vi "Information.vi"(8 "error in (no error)":errorcluster, 9 "Context":T1, 10 "Information":refnum<class "Information.lvclass">, 11 "Process Controller in":refnum<class "Process Controller.lvclass">) -> (0 "error out":errorcluster, 3 "Process Controller out":refnum<class "Process Controller.lvclass">)   [LabVIEW 2021, in "Process Controller.lvclass"]
uses:
  Process Controller.lvclass
  Publish-Subscribe/Interfaces/Information/Information.lvclass
  Publish-Subscribe/Context.ctl
  NHMFL_Core/Libraries/Instruments/Results/Acquired Result/Acquired Result.lvclass
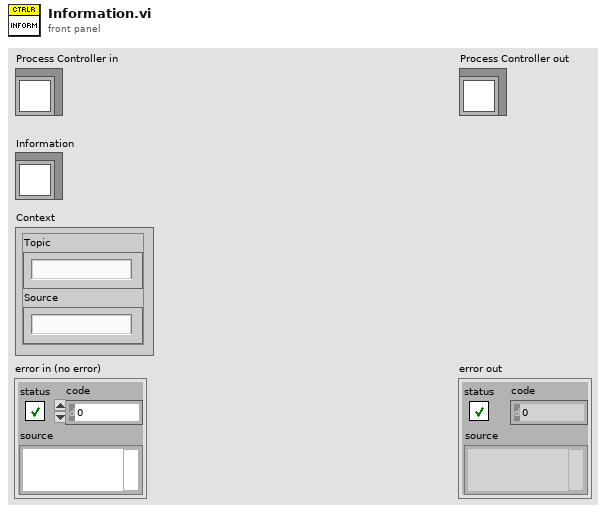
[diagram p1: front panel]
types:
  T1 = typedef "Context.ctl" = cluster{"Topic":string, "Source":string}
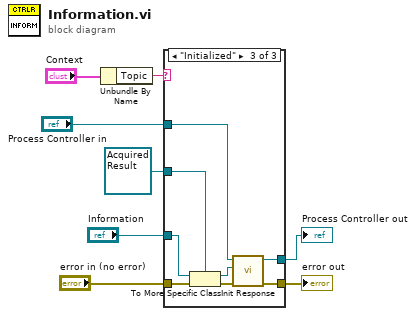
[diagram p0: block diagram]
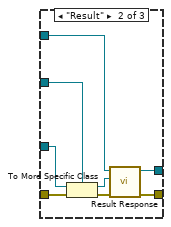
[diagram p3: hidden frame]
diagram:
  n1 = Unbundle By Name("Context") -> ("Topic"=w1:string)
  n2 = case shown="\"Initialized\"" w1 {
    tunnel: "Process Controller in" -> [w9 w18 w26]
    tunnel: refnum<class "Acquired Result.lvclass"> refnum ("Acquired Result") -> [_ w17 w25]
    tunnel: "Information" -> [_ w16 w24]
    tunnel: "error in (no error)" -> [w10 w14 w22]
    tunnel: [w10 w12 w20] -> w3
    tunnel: [w9 w11 w19] -> w2
    frame "", Default {
    }
    frame "Result" {
      n3 = To More Specific Class(target class=w17, reference=w16, error in=w14) -> (specific class reference=w15:refnum<class "Acquired Result.lvclass">, error out=w13:errorcluster)
      n4 = call-dynamic "Result Response.vi"("error in (no error)"=w13, "Acquired Result"=w15, "Measure Controller in"=w18) -> ("error out"=w12:errorcluster, "Measure Controller out"=w11:refnum<class "Process Controller.lvclass">)  [unwired: 7 in]
    }
    frame "Initialized" {
      n5 = To More Specific Class(target class=w25, reference=w24, error in=w22) -> (specific class reference=w23:refnum<class "Acquired Result.lvclass">, error out=w21:errorcluster)
      n6 = call-dynamic "Init Response.vi"("error in (no error)"=w21, "Result"=w23, "Measure Controller in"=w26) -> ("error out"=w20:errorcluster, "Measure Controller out"=w19:refnum<class "Process Controller.lvclass">)  [unwired: 7 in]
    }
  }
  "error out" <- w3
  "Process Controller out" <- w2
